vi "write(sub).vi"(0 "resourcein":refnum<visa-resource-name>, 1 "readdelay":u32=500, 2 "writestring":string="R0003", 3 "errorin":errorcluster, 4 "payload":string="R0003") -> (5 "resourceout":refnum<visa-resource-name>, 6 "errorout":errorcluster)   [LabVIEW 2015]
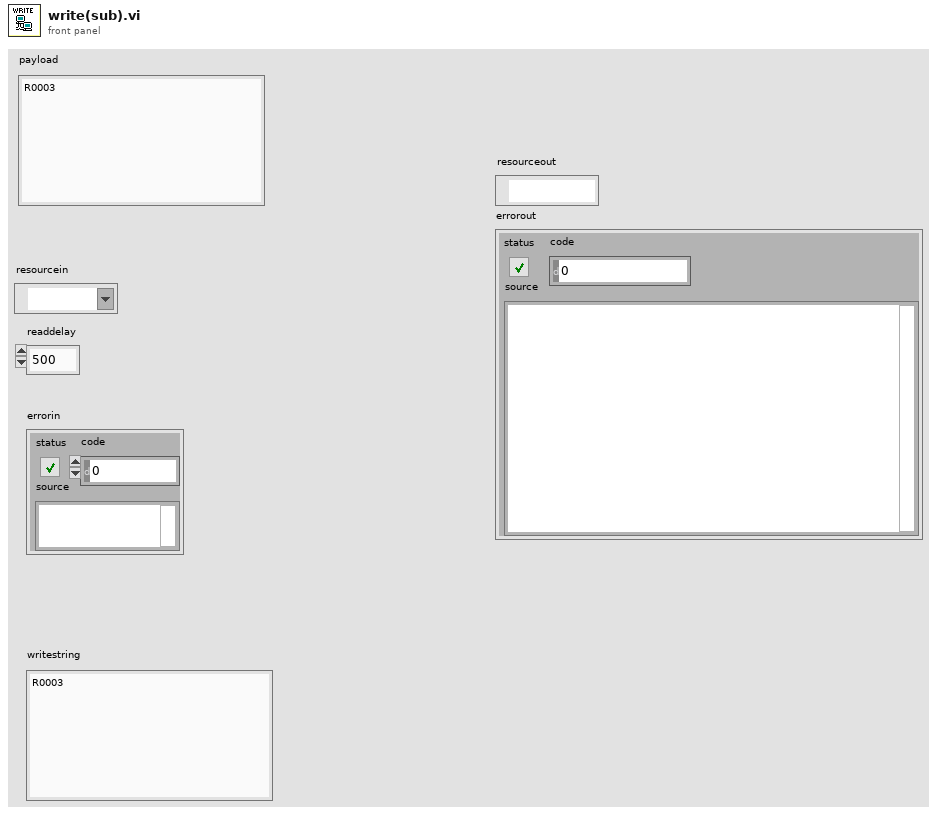
[diagram p1: front panel]
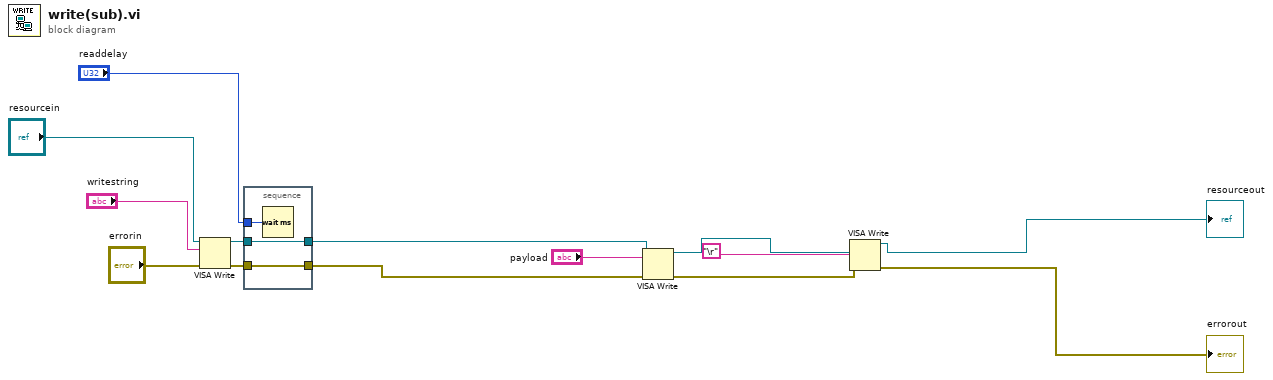
[diagram p0: block diagram]
diagram:
  n1 = VISA Write(VISA resource name="resourcein", write buffer="writestring", error in (no error)="errorin") -> (VISA resource name out=w10:refnum<visa-resource-name>, error out=w9:errorcluster)  [unwired: 1 out]
  n2 = stacked-sequence {
    tunnel: w9 -> [w17]
    tunnel: [w17] -> w7
    tunnel: w10 -> [w16]
    tunnel: [w16] -> w8
    tunnel: "readdelay" -> [w15]
    frame #0 {
      n3 = Wait (ms)(milliseconds to wait=w15) -> ()  [unwired: 1 out]
    }
  }
  n4 = VISA Write(VISA resource name=w8, write buffer="payload", error in (no error)=w7) -> (VISA resource name out=w4:refnum<visa-resource-name>, error out=w3:errorcluster)  [unwired: 1 out]
  n5 = VISA Write(VISA resource name=w4, write buffer="\r", error in (no error)=w3) -> (VISA resource name out=→"resourceout":refnum<visa-resource-name>, error out=→"errorout":errorcluster)  [unwired: 1 out]
